vi "Experiment header-Gen user name stamp file.vi"(8 "error in (no error)":errorcluster, 11 "Experiment data folder path":path) -> (0 "error out":errorcluster)   [LabVIEW 2017]
uses:
  User profiles code/Globals/gl_UsrProfiles globals.vi
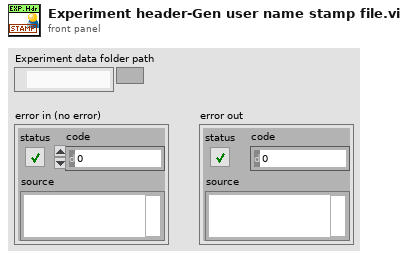
[diagram p1: front panel]
types:
  T1 = enum16{"open", "replace", "create", "open or create", "replace or create", "replace or create with confirmation"}
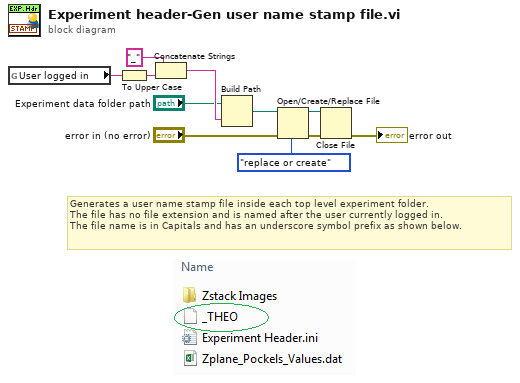
[diagram p0: block diagram]
diagram:
  # "Generates a user name stamp file inside each top level experiment folder.\nThe file has no file extension and is named after the user currently logged in.\nThe file name is in Capitals and has an underscore symbol prefix as shown below."
  n1 = global read "gl_UsrProfiles globals.vi" "User logged in"() -> (w8:string)
  n2 = To Upper Case(1:w8) -> (0:w9:string)
  n3 = Concatenate Strings("_" ("string"), w9) -> (w3:string)
  n4 = Build Path(base path="Experiment data folder path", name or relative path=w3) -> (appended path=w4:path)
  n5 = Open/Create/Replace File(file path (use dialog)=w4, error in="error in (no error)", operation (0:open)=T1."replace or create") -> (refnum out=w5:refnum<file>, error out=w6:errorcluster)  [unwired: 3 in, 1 out]
  n6 = Close File(refnum=w5, error in=w6) -> (error out=→"error out":errorcluster)  [unwired: 1 out]
